vi "ProjectVersionCheck_Global_OnCommand.vi"(10 "Command ID":string, 11 "Object":T1) -> ()   [LabVIEW 2015]
doc: "#translatableVI"
uses:
  <resource>/Framework/Providers/API/ItemRef.ctl
  <vilib>/Platform/browser.llb/Open URL in Default Browser (string).vi
panel:
  out "error out":errorcluster
  in  "error in":errorcluster
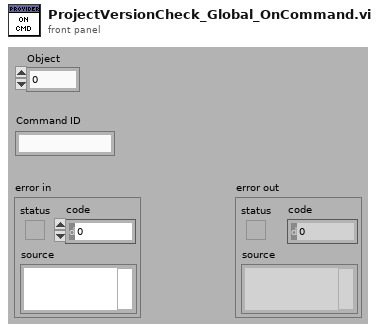
[diagram p1: front panel]
types:
  T1 = typedef "ItemRef.ctl" = u64
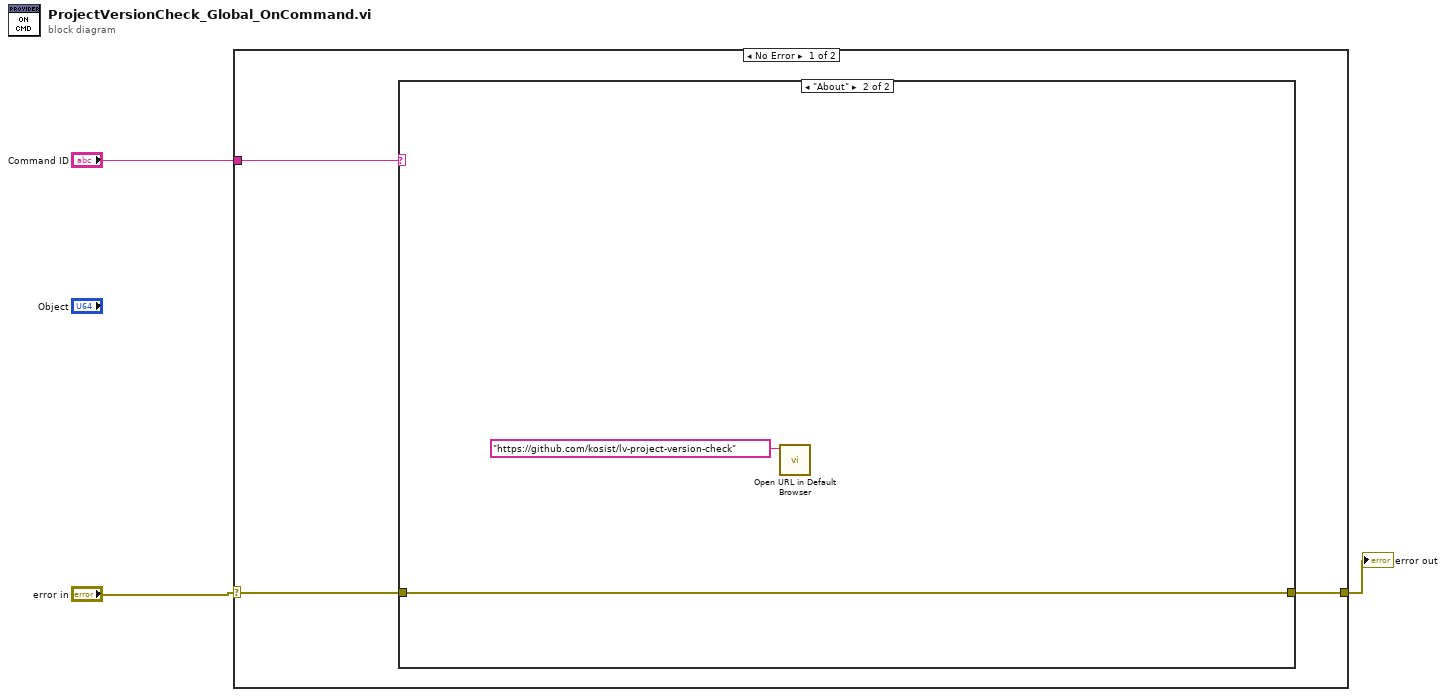
[diagram p0: block diagram]
diagram:
  n1 = case shown="No Error" "error in" {
    selector: "error in" -> [w4 w10]
    tunnel: "Command ID" -> [w6 _]
    tunnel: [w5 w10] -> w3
    frame No Error {
      n2 = case shown="\"About\"" w6 {
        tunnel: [w7 w9] -> w5
        tunnel: w4 -> [w7 w9]
        frame Default {
        }
        frame "About" {
          n3 = call-poly <vilib>:"Open URL in Default Browser.vi"("URL"="https://github.com/kosist/lv-project-version-check") -> ()  [unwired: 5 in, 2 out]
        }
      }
    }
    frame Error {
    }
  }
  "error out" <- w3
